vi "init_cards.vi"(8 "error in (no error)":errorcluster, 11 "VISA Refnum in":refnum<visa-resource-name>) -> (0 "error out":errorcluster, 1 "init ok?":bool, 2 "read buffer":string, 3 "VISA Refnum out":refnum<visa-resource-name>)   [LabVIEW 2018]
doc: "the Conrad Relais Cards are initialized, meaning that each card is assigned a number. Card 1 = Number 1, Card 2 = Number 2,...\n\nThe command \"1\" is send to the cards. only one command needs to be send no matter how many cards are installed. The card controllers deal with the commands themselfes."
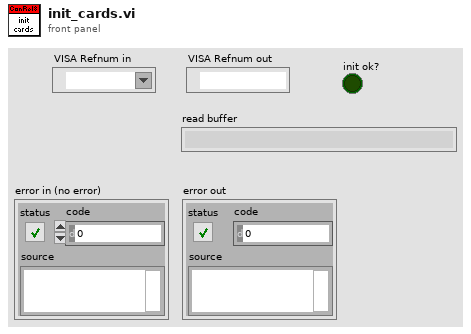
[diagram p1: front panel]
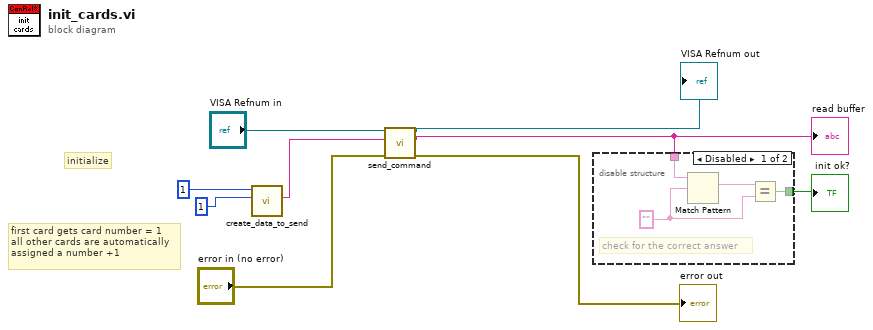
[diagram p0: block diagram]
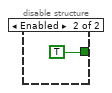
[diagram p2: hidden frame]
diagram:
  # "first card gets card number = 1\nall other cards are automatically\nassigned a number +1"
  # "initialize"
  n1 = call "create_data_to_send.vi"("address"=u8 1, "command"=u8 1) -> ("send string"=w1:string)  [unwired: 6 in, 3 out]
  n2 = call "send_command.vi"("error in (no error)"="error in (no error)", "command"=w1, "VISA Refnum in"="VISA Refnum in") -> ("error out"=→"error out":errorcluster, "return string"=w4:string, "VISA resource name out"=→"VISA Refnum out":refnum<visa-resource-name>)  [unwired: 5 in, 1 out]
  "read buffer" <- w4
  n3 = disable-structure shown="Disabled" {
    disable-tunnel: w4 -> [w11 _]
    disable-tunnel: [w10 TRUE] -> w2
    frame Disabled {
      w12 = "" ("regular expression")
      # "check for the correct answer"
      n4 = Match Pattern(string=w11, regular expression=w12) -> (match substring=w13:string)  [unwired: 1 in, 3 out]
      n5 = Equal?(x=w13, y=w12) -> (x = y?=w10:bool)
    }
    frame Enabled {
    }
  }
  "init ok?" <- w2
